vi "Boolean operators.vi"() -> ()   [LabVIEW 2019]
panel:
  out "A .implies. B?":bool
  out ".not. (A .Aor. B)?":bool
  out ".not. (A .and. B)?":bool
  out ".not. A?":bool
  out "A .Aor. B?":bool
  out "A .or. B?":bool
  out "A .and. B?":bool
  in  "B":bool
  in  "A":bool
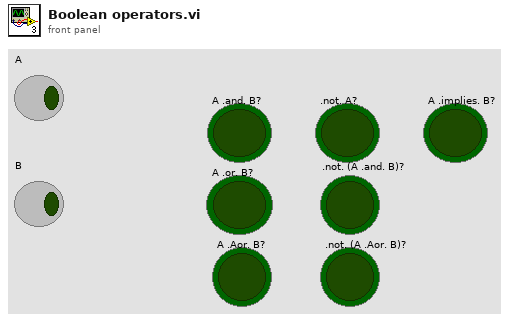
[diagram p1: front panel]
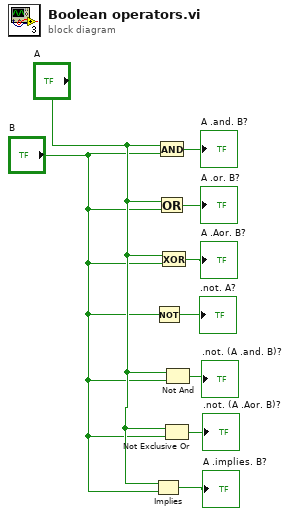
[diagram p0: block diagram]
diagram:
  n1 = Implies(1:"B", 2:"A") -> (0:→"A .implies. B?":bool)
  n2 = Not(x="B") -> (.not. x?=→".not. A?":bool)
  n3 = And(x="A", y="B") -> (x .and. y?=→"A .and. B?":bool)
  n4 = Or(x="A", y="B") -> (x .or. y?=→"A .or. B?":bool)
  n5 = Exclusive Or(1:"B", 2:"A") -> (0:→"A .Aor. B?":bool)
  n6 = Not Exclusive Or(1:"B", 2:"A") -> (0:→".not. (A .Aor. B)?":bool)
  n7 = Not And(1:"B", 2:"A") -> (0:→".not. (A .and. B)?":bool)
